vi "TeddingtonParser.vi"(11 "webpage":string) -> (0 "timeOfValue":dbl, 1 "Time Stamp GMT":timestamp, 2 "SeaLevelPressure":dbl, 3 "NotFound":bool)   [LabVIEW 2011]
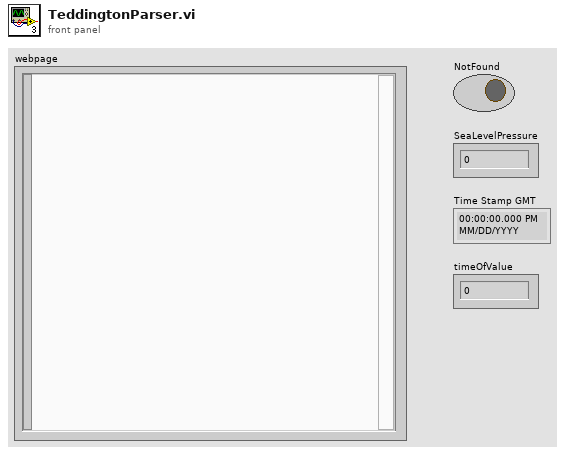
[diagram p1: front panel]
types:
  T1 = cluster{"second":i32, "minute":i32, "hour":i32, "day of month":i32, "month":i32, "year":i32, "day of week":i32, "day of year":i32, "is DST":i32}
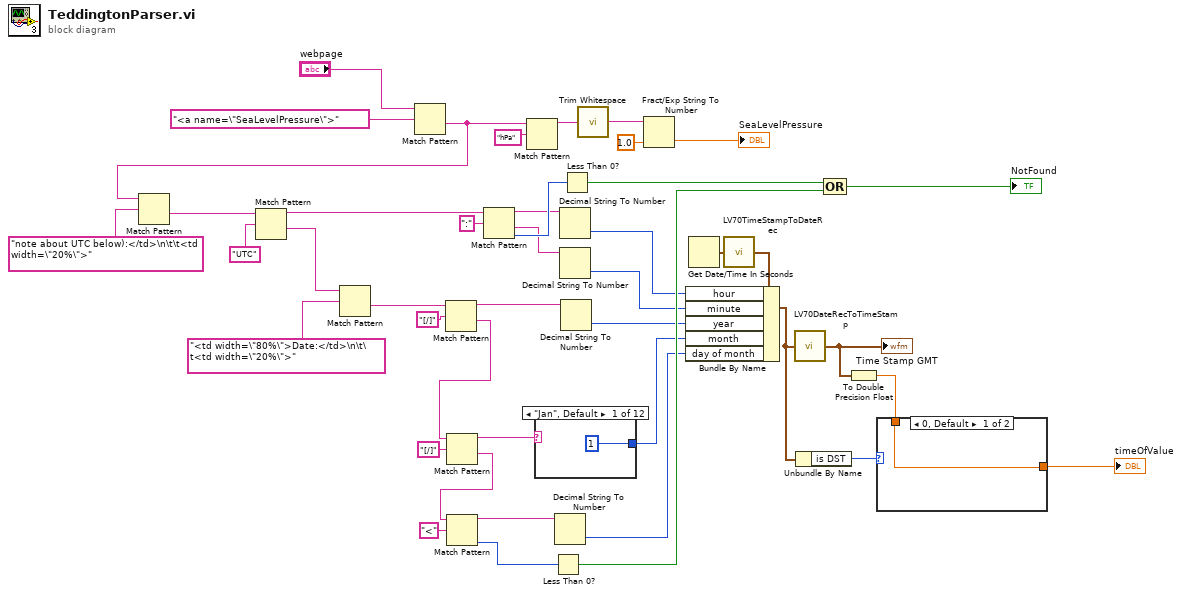
[diagram p0: block diagram]
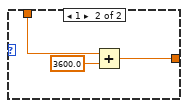
[diagram p2: hidden frame]
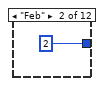
[diagram p3: hidden frame]
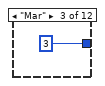
[diagram p4: hidden frame]
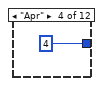
[diagram p5: hidden frame]
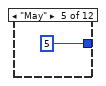
[diagram p6: hidden frame]
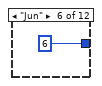
[diagram p7: hidden frame]
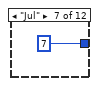
[diagram p8: hidden frame]
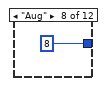
[diagram p9: hidden frame]
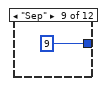
[diagram p10: hidden frame]
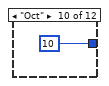
[diagram p11: hidden frame]
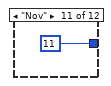
[diagram p12: hidden frame]
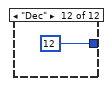
[diagram p13: hidden frame]
diagram:
  n1 = Match Pattern(string="webpage", regular expression="<a name=\"SeaLevelPressure\">") -> (after substring=w38:string)  [unwired: 4 out]
  n2 = Match Pattern(string=w38, regular expression="note about UTC below):</td>\n\t\t<td width=\"20%\">") -> (after substring=w6:string)  [unwired: 4 out]
  n3 = Match Pattern(string=w6, regular expression="UTC") -> (before substring=w11:string, after substring=w25:string)  [unwired: 3 out]
  n4 = Match Pattern(string=w25, regular expression="<td width=\"80%\">Date:</td>\n\t\t<td width=\"20%\">") -> (after substring=w13:string)  [unwired: 4 out]
  n5 = Match Pattern(string=w13, regular expression="[/]") -> (before substring=w17:string, after substring=w18:string)  [unwired: 3 out]
  n6 = Match Pattern(string=w18, regular expression="[/]") -> (before substring=w20:string, after substring=w19:string)  [unwired: 3 out]
  n7 = Match Pattern(string=w19, regular expression="<") -> (before substring=w22:string, offset past match=w31:i32)  [unwired: 3 out]
  n8 = Match Pattern(string=w11, regular expression=":") -> (before substring=w7:string, after substring=w8:string, offset past match=w32:i32)  [unwired: 2 out]
  n9 = Match Pattern(string=w38, regular expression="hPa") -> (before substring=w42:string)  [unwired: 4 out]
  n10 = case shown="\"Jan\", Default" w20 {
    tunnel: [1 ("month") 2 ("month") 3 ("month") 4 ("month") 5 ("month") 6 ("month") 7 ("month") 8 ("month") 9 ("month") 10 ("month") 11 ("month") 12 ("month")] -> w21
    frame "Jan", Default {
    }
    frame "Feb" {
    }
    frame "Mar" {
    }
    frame "Apr" {
    }
    frame "May" {
    }
    frame "Jun" {
    }
    frame "Jul" {
    }
    frame "Aug" {
    }
    frame "Sep" {
    }
    frame "Oct" {
    }
    frame "Nov" {
    }
    frame "Dec" {
    }
  }
  n11 = Less Than 0?(x=w31) -> (x < 0?=w36:bool)
  n12 = Decimal String To Number(string=w22) -> (number=w23:i32)  [unwired: 3 out]
  n13 = Decimal String To Number(string=w7) -> (number=w10:i32)  [unwired: 3 out]
  n14 = Decimal String To Number(string=w8) -> (number=w9:i32)  [unwired: 3 out]
  n15 = Decimal String To Number(string=w17) -> (number=w16:i32)  [unwired: 3 out]
  n16 = Less Than 0?(x=w32) -> (x < 0?=w37:bool)
  n17 = call <vilib>:"Trim Whitespace.vi"("string"=w42) -> ("trimmed string"=w35:string)  [unwired: 1 in]
  n18 = Fract/Exp String To Number(string=w35, default (0 dbl)=1.0 ("default (0 DBL)")) -> (number=→"SeaLevelPressure":dbl)  [unwired: 3 out]
  n19 = Get Date/Time In Seconds() -> (seconds since 1Jan1904=w41:timestamp)
  n20 = call <vilib>:"LV70TimeStampToDateRec.vi"("time stamp"=w41) -> ("date time rec"=w26:T1)
  n21 = Bundle By Name(cluster=w26, "hour"=w10, "minute"=w9, "year"=w16, "month"=w21, "day of month"=w23) -> (w28:T1)
  n22 = call <vilib>:"LV70DateRecToTimeStamp.vi"("date time rec"=w28) -> ("Time Stamp"=w27:timestamp)
  "Time Stamp GMT" <- w27
  n23 = Unbundle By Name(w28) -> ("is DST"=w29:i32)
  n24 = Compound Arithmetic op=OR(w37, w36) -> (→"NotFound":bool)
  n25 = To Double Precision Float(number=w27) -> (double precision float=w30:dbl)
  n26 = case shown="0, Default" w29 {
    tunnel: w30 -> [w56 w59]
    tunnel: [w56 w57] -> w40
    frame 0, Default {
    }
    frame 1 {
      n27 = Add(x=w59, y=3600.0) -> (x+y=w57:dbl)
    }
  }
  "timeOfValue" <- w40
